vi "sub vi4.vi"() -> ()   [LabVIEW 2023]
panel:
  out "Numeric 2":dbl
  in  "Numeric 4":dbl
  out "Numeric":dbl
  in  "Numeric 3":dbl
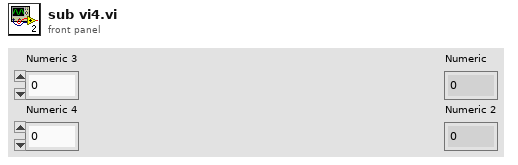
[diagram p1: front panel]
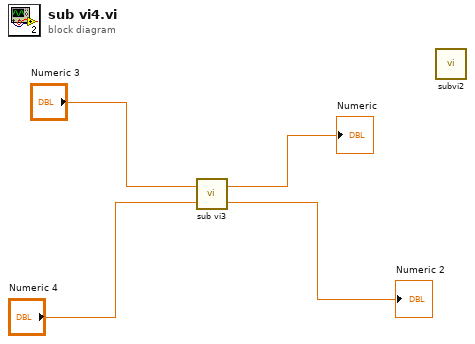
[diagram p0: block diagram]
diagram:
  n1 = call "sub vi3.vi"("Numeric 4"="Numeric 4", "Numeric 3"="Numeric 3") -> ("Numeric 2"=→"Numeric 2":dbl, "Numeric"=→"Numeric":dbl)
  n2 = call "subvi2.vi"() -> ()  [unwired: 2 in, 2 out]
